vi "Do.vi"(8 "error in (no error)":errorcluster, 10 "Actor in":refnum<class "Actor.lvclass">, 11 "PrepareAndSendStartAcq Msg":refnum<class "PrepareAndSendStartAcq Msg.lvclass">) -> (0 "error out":errorcluster, 2 "Actor out":refnum<class "Actor.lvclass">)   [LabVIEW 2020, in "CameraController.lvlib" / "PrepareAndSendStartAcq Msg.lvclass"]
doc: "This VI delivers the message to the actor by calling the appropriate method(s) on the actor."
uses:
  PrepareAndSendStartAcq Msg.lvclass
  <vilib>/ActorFramework/Actor/Actor.lvclass
  PrepareAndSendStartAcq Msg.lvclass/PrepareAndSendStartAcq Msg.ctl
  Prime95BCameraController/CameraController.lvclass
  C:/Program Files/National Instruments/LabVIEW 2020/vi.lib/ActorFramework/Actor/Actor.lvclass
  9ef47adc-f318-494c-9b8b-6df3216d6863.vi
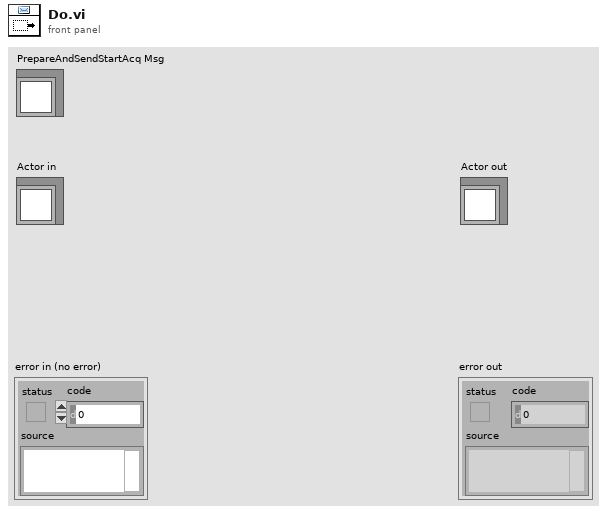
[diagram p1: front panel]
types:
  T1 = typedef "Camera_Prime95B.lvlib/Camera_Prime95B.lvclass/Camera Status.ctl" = i32
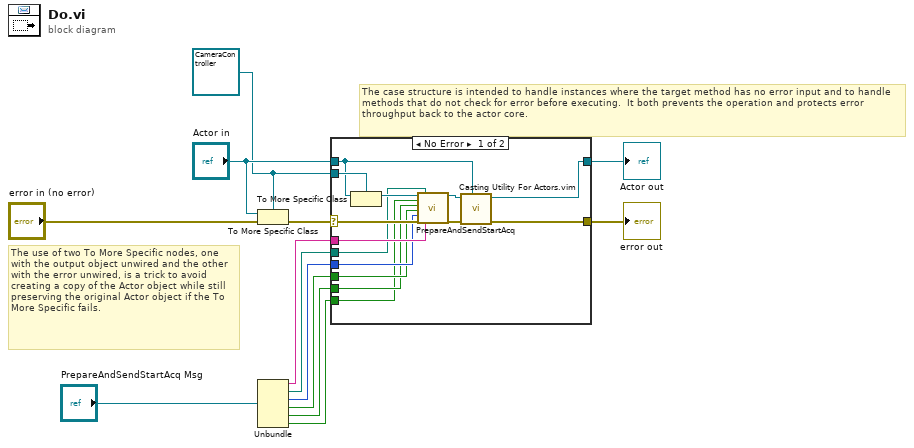
[diagram p0: block diagram]
diagram:
  w7 = refnum<class "CameraController.lvclass"> refnum ("Actor in")
  # "The use of two To More Specific nodes, one with the output object unwired and the other with the error unwired, is a trick to avoid creating a copy of the Actor object while still preserving the original Actor object if the To More Specific fails."
  # "The case structure is intended to handle instances where the target method has no error input and to handle methods that do not check for error before executing.  It both prevents the operation and protects error throughput back to the actor core."
  n1 = To More Specific Class(target class=w7, reference="Actor in", error in="error in (no error)") -> (error out=w11:errorcluster)  [unwired: 1 out]
  n2 = Unbundle("PrepareAndSendStartAcq Msg") -> (w6:string, w5:path, w4:T1, w3:bool, w2:bool, w1:bool)
  n3 = case shown="No Error" w11 {
    selector: w11 -> [w27 w29]
    tunnel: [w21 w29] -> w10
    tunnel: [w22 w28] -> w9
    tunnel: "Actor in" -> [w24 w28]
    tunnel: w7 -> [w25 _]
    tunnel: w6 -> [w19 _]
    tunnel: w5 -> [w18 _]
    tunnel: w4 -> [w17 _]
    tunnel: w3 -> [w16 _]
    tunnel: w2 -> [w15 _]
    tunnel: w1 -> [w14 _]
    frame No Error {
      n4 = To More Specific Class(target class=w25, reference=w24) -> (specific class reference=w26:refnum<class "CameraController.lvclass">)  [unwired: 1 in, 1 out]
      n5 = call-dynamic "PrepareAndSendStartAcq.vi"("CameraController in"=w26, "SingleStack?"=w14, "StreamToDisk?"=w15, "Alert when finish?"=w16, "Mode"=w17, "error in (no error)"=w27, "Save Path"=w18, "File Suffix"=w19) -> ("CameraController out"=w23:refnum<class "CameraController.lvclass">, "error out"=w20:errorcluster)  [unwired: 10 in]
      n6 = call "Casting Utility For Actors.vim"("type"=w24, "error in (no error)"=w20, "Actor in"=w23) -> ("error out"=w21:errorcluster, "Actor out"=w22:refnum<class "Actor.lvclass">)  [unwired: 7 in]
    }
    frame Error {
      # "If type check fails, pass the original object out again."
    }
  }
  "error out" <- w10
  "Actor out" <- w9
